vi "Generate Icon.vi"(6 "Access":enum16{"Read", "Write", "R/W"}(ring)=enum."Write", 8 "error in (no error)":errorcluster, 9 "Body":T1={"Line 1 text"="    ", "Line 2 text"="GEN", "Line 3 text"="ICON", "Body text color"=2171169}, 10 "Header":T3={"Header text"="TEST", "Header colors (black, white)"={"Border"=0, "Background"=16730898}, "Header text color"=16777226}, 11 "VI ref":refnum<vi>) -> (0 "error out":errorcluster, 3 "VI ref out":refnum<vi>)   [LabVIEW 2018]
doc: "Generates icon and text for new VI accessors."
uses:
  <vilib>/LabVIEW Icon API/API_Rectangle Colors.ctl
  <vilib>/LabVIEW Icon API/API_Rectangle Dimension.ctl
  <vilib>/LabVIEW Icon API/API_Test Settings.ctl
  <vilib>/LabVIEW Icon API/lv_icon/Controls/Alignment.ctl
  <vilib>/LabVIEW Icon API/API_Text Colors.ctl
  <vilib>/LabVIEW Icon API/API_Text.ctl
  <vilib>/LabVIEW Icon API/API_User Layer Data.ctl
  <vilib>/Utility/miscctls.llb/LVPoint32TypeDef.ctl
  <vilib>/picture/picture.llb/imagedata.ctl
  <vilib>/Utility/error.llb/Clear Errors.vi
  <userlib>/nLight Error Handling/Log any errors.vi
  <vilib>/LabVIEW Icon API/LabVIEW Icon API.lvlib
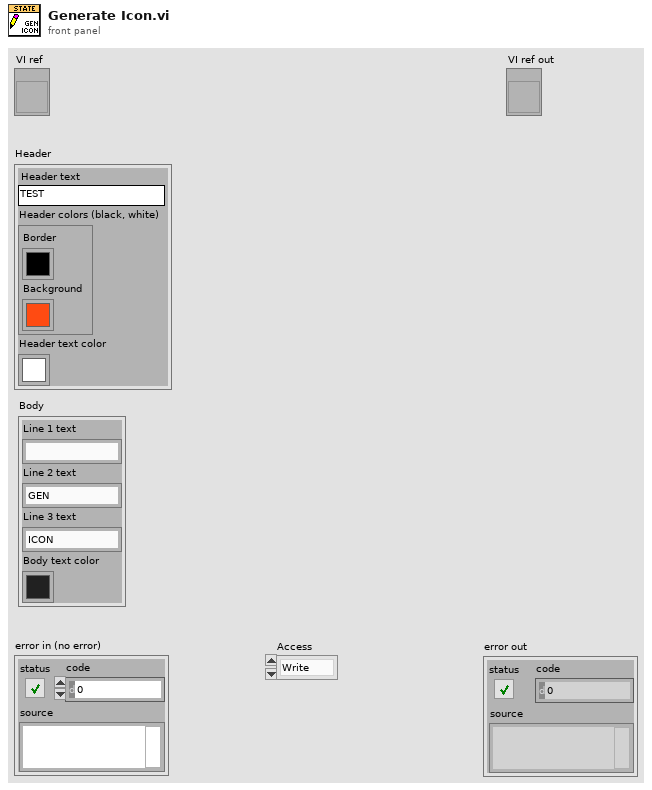
[diagram p1: front panel]
types:
  T1 = cluster{"Line 1 text":string, "Line 2 text":string, "Line 3 text":string, "Body text color":u32}
  T2 = typedef "LabVIEW Icon API.lvlib/API_Rectangle Colors.ctl" = cluster{"Border":u32, "Background":u32}
  T3 = cluster{"Header text":string, "Header colors (black, white)":T2, "Header text color":u32}
  T4 = typedef "Alignment.ctl" = u16
  T5 = typedef "LabVIEW Icon API.lvlib/API_Text.ctl" = cluster{"Line 1 text":string, "Line 2 text":string, "Line 3 text":string, "Line 4 text":string}
  T6 = typedef "LabVIEW Icon API.lvlib/API_Test Settings.ctl" = cluster{"Font":string, "Alignment":T4, "Size":u8, "Center text":bool, "Capitalize text":bool, "Text color":T7}
  T7 = typedef "LabVIEW Icon API.lvlib/API_Text Colors.ctl" = cluster{"Line 1 color":u32, "Line 2 color":u32, "Line 3 color":u32, "Line 4 color":u32}
  T8 = typedef "LabVIEW Icon API.lvlib/API_Rectangle Dimension.ctl" = cluster{"Width":i16, "Height":i16}
  T9 = typedef "imagedata.ctl" = cluster{"image type":i32, "image depth":i32, "image":u8[], "mask":u8[], "colors":u32[], "Rectangle":cluster{"left":i16, "top":i16, "right":i16, "bottom":i16}}
  T10 = typedef "LabVIEW Icon API.lvlib/API_User Layer Data.ctl" = cluster{"Layer name":string, "Origin":T11, "Icon image data":T9}
  T11 = typedef "LVPoint32TypeDef.ctl" = cluster{"Horizontal":i32, "Vertical":i32}
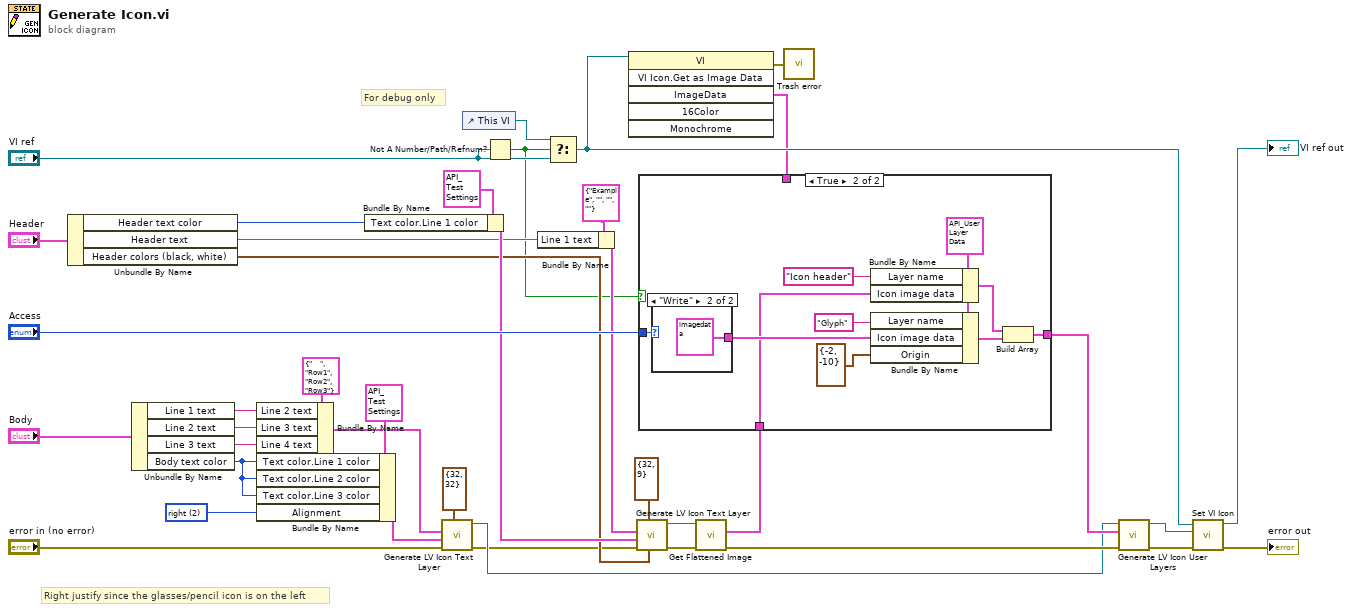
[diagram p0: block diagram]
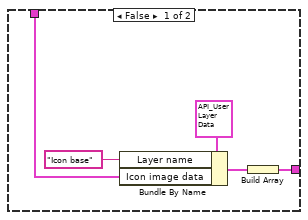
[diagram p2: hidden frame]
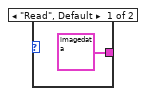
[diagram p3: hidden frame]
diagram:
  w2 = T4 2 items=["left", "center", "right"] ("Alignment")
  # "Right justify since the glasses/pencil icon is on the left"
  # "For debug only"
  n1 = Unbundle By Name("Header") -> ("Header text color"=w20:u32, "Header text"=w19:string, "Header colors (black, white)"=w18:T2)
  n2 = Unbundle By Name("Body") -> ("Line 1 text"=w11:string, "Line 2 text"=w10:string, "Line 3 text"=w9:string, "Body text color"=w16:u32)
  n3 = Bundle By Name(cluster=T5 {"Line 1 text"="    ", "Line 2 text"="Row1", "Line 3 text"="Row2", "Line 4 text"="Row3"} ("Body text"), "Line 2 text"=w11, "Line 3 text"=w10, "Line 4 text"=w9) -> (w12:T5)
  n4 = Bundle By Name(cluster=T6 {"Font"="Small Fonts", "Alignment"=2, "Size"=9, "Center text"=TRUE, "Capitalize text"=TRUE, "Text color"={"Line 1 color"=0, "Line 2 color"=0, "Line 3 color"=0, "Line 4 color"=0}} ("Text settings"), "Text color.Line 1 color"=w16, "Text color.Line 2 color"=w16, "Text color.Line 3 color"=w16, "Alignment"=w2) -> (w24:T6)
  n5 = Bundle By Name(cluster=T6 {"Font"="Small Fonts", "Alignment"=1, "Size"=8, "Center text"=TRUE, "Capitalize text"=TRUE, "Text color"={"Line 1 color"=0, "Line 2 color"=0, "Line 3 color"=0, "Line 4 color"=0}} ("Text settings"), "Text color.Line 1 color"=w20) -> (w26:T6)
  n6 = call <vilib>:"Generate LV Icon Text Layer.vi"("Rectangle dimension (32,32)"=T8 {"Width"=32, "Height"=32}, "error in (no error)"="error in (no error)", "Text settings"=w24, "Text"=w12) -> ("error out"=w14:errorcluster, "Icon out"=w15:refnum<class "Icon.lvclass">)  [unwired: 6 in]
  n7 = control-ref of="This VI"() -> (w7:refnum<vi>)
  n8 = Not A Number/Path/Refnum?(number/path/refnum="VI ref") -> (NaN/Path/Refnum?=w3:bool)
  n9 = Bundle By Name(cluster=T5 {"Line 1 text"="Example", "Line 2 text"="", "Line 3 text"="", "Line 4 text"=""} ("Text"), "Line 1 text"=w19) -> (w28:T5)
  n10 = Select(t=w7, s=w3, f="VI ref") -> (s? t:f=w5:refnum<vi>)
  n11 = invoke class="VI" method="VI Icon.Get as Image Data"(reference=w5) -> (error out=w1:errorcluster, "ImageData"=w4:T9)  [unwired: 5 in, 4 out]
  n12 = call <vilib>:"Generate LV Icon Text Layer.vi"("Rectangle colors (black, white)"=w18, "Rectangle dimension (32,32)"=T8 {"Width"=32, "Height"=9}, "error in (no error)"=w14, "Text settings"=w26, "Text"=w28) -> ("error out"=w30:errorcluster, "Icon out"=w32:refnum<class "Icon.lvclass">)  [unwired: 5 in]
  n13 = call <vilib>:"Get Flattened Image.vi"("error in (no error)"=w30, "lv_icon.lvlib:Icon.lvclass in"=w32) -> ("error out"=w29:errorcluster, "Color Image"=w33:T9)  [unwired: 6 in, 2 out]
  n14 = case shown="True" w3 {
    tunnel: [w41 w53] -> w38
    tunnel: "Access" -> [_ w52]
    tunnel: w33 -> [_ w50]
    tunnel: w4 -> [w40 _]
    frame False {
      n15 = Bundle By Name(cluster=T10 {"Layer name"="", "Origin"={"Horizontal"=0, "Vertical"=0}, "Icon image data"={"image type"=0, "image depth"=0, "image"=[], "mask"=[], "colors"=[], "Rectangle"={"left"=0, "top"=0, "right"=0, "bottom"=0}}} ("User layer"), "Layer name"="Icon base", "Icon image data"=w40) -> (w42:T10)
      n16 = Build Array(w42) -> (w41:T10[])
    }
    frame True {
      w46 = T10 {"Layer name"="", "Origin"={"Horizontal"=0, "Vertical"=0}, "Icon image data"={"image type"=0, "image depth"=0, "image"=[], "mask"=[], "colors"=[], "Rectangle"={"left"=0, "top"=0, "right"=0, "bottom"=0}}} ("User layer")
      n17 = case shown="\"Write\"" w52 {
        tunnel: [T9 {"image type"=0, "image depth"=24, "image"=[255, 255, 255, 255, 255, 255, 255, 255, 255, 255, 255, 255, 255, 255, 255, 0, 0, 0, 0, 0, 0, 255, 255, 255, 255, 255, 255, 255, 255, 255, 255, 255, 255, 255, 255, 255, 255, 255, 255, 0, 0, 0, 0, 0, 0, 255, 255, 255, 255, 255, 255, 255, 255, 255, 255, 255, 255, 255, 255, 255, 0, 0, 0, 255, 255, 255, 255, 255, 255, 0, 0, 0, 255, 255, 255, 255, 255, 255, 255, 255, 255, 255, 255, 255, 0, 0, 0, 255, 255, 255, 255, 255, 255, 0, 0, 0, 255, 255, 255, 255, 255, 255, 255, 255, 255, 0, 0, 0, 255, 255, 255, 255, 255, 255, 255, 255, 255, 0, 0, 0, 255, 255, 255, 255, 255, 255, 255, 255, 255, 0, 0, 0, 255, 255, 255, 255, 255, 255, 255, 255, 255, 0, 0, 0, 255, 255, 255, 255, 255, 255, 0, 0, 0, 0, 0, 0, 255, 255, 255, 255, 255, 255, 255, 255, 255, 255, 255, 255, 255, 255, 255, 255, 255, 255, 0, 0, 0, 0, 0, 0, 255, 255, 255, 255, 255, 255, 255, 255, 255, 255, 255, 255, 255, 255, 255, 0, 0, 0, 255, 255, 255, 255, 255, 255, 0, 0, 0, 255, 255, 255, 0, 0, 0, 0, 0, 0, 255, 255, 255, 0, 0, 0, 255, 255, 255, 0, 255, 255, 0, 0, 0, 255, 255, 255, 255, 255, 255, 255, 255, 255, 0, 0, 0, 255, 255, 255, 255, 255, 255, 0, 255, 255, 0, 255, 255, 0, 0, 0, 255, 255, 255, 255, 255, 255, 0, 0, 0, 255, 255, 255, 255, 255, 255, 255, 255, 255, 0, 255, 255, 0, 0, 0, 255, 255, 255, 255, 255, 255, 0, 0, 0, 0, 255, 255, 255, 255, 255, 0, 255, 255, 0, 214, 214, 0, 0, 0, 255, 255, 255, 255, 255, 255, 0, 0, 0, 0, 255, 255, 255, 255, 255, 0, 255, 255, 0, 214, 214, 0, 0, 0, 255, 255, 255, 255, 255, 255, 255, 255, 255, 0, 0, 0, 0, 255, 255, 0, 255, 255, 0, 0, 0, 255, 255, 255, 255, 255, 255, 255, 255, 255, 255, 255, 255, 0, 0, 0, 0, 255, 255, 0, 214, 214, 0, 0, 0, 255, 255, 255, 255, 255, 255, 255, 255, 255, 255, 255, 255, 255, 255, 255, 0, 0, 0, 0, 0, 0, 255, 255, 255, 255, 255, 255, 255, 255, 255, 255, 255, 255, 255, 255, 255, 255, 255, 255, 0, 0, 0, 0, 0, 0, 255, 255, 255, 255, 255, 255, 255, 255, 255, 255, 255, 255, 255, 255, 255, 255, 255, 255, 255, 255, 255, 255, 255, 255, 255, 255, 255, 255, 255, 255, 255, 255, 255, 255, 255, 255, 255, 255, 255, 255, 255, 255, 255, 255, 255, 255, 255, 255, 255, 255, 255, 255, 255, 255, 255, 255, 255, 255, 255, 255, 255, 255, 255, 255, 255, 255, 255, 255, 255, 255, 255, 255, 255, 255, 255, 255, 255, 255, 255, 255, 255, 255, 255, 255, 255, 255, 255, 255, 255, 255, 255, 255, 255, 255, 255, 255, 255, 255, 255, 255, 255, 255, 255, 255, 255, 255, 255, 255, 255, 255, 255, 255, 255, 255, 255, 255, 255, 255, 255, 255, 255, 255, 255, 255, 255, 255, 255, 255, 255, 255, 255, 255, 255, 255, 255, 255, 255, 255, 255, 255, 255, 255, 255, 255, 255, 255, 255, 255, 255, 255, 255, 255, 255, 255, 255, 255, 255, 255, 255, 255, 255, 255, 255, 255, 255, 255, 255, 255, 255, 255, 255, 255, 255, 255, 255, 255, 255, 255, 255, 255, 255, 255, 255, 255, 255, 255, 255, 255, 255, 255, 255, 255, 255, 255, 255, 255, 255, 255, 255, 255, 255, 255, 255, 255], "mask"=[], "colors"=[], "Rectangle"={"left"=0, "top"=0, "right"=16, "bottom"=13}} ("image subset") T9 {"image type"=0, "image depth"=8, "image"=[0, 0, 0, 0, 1, 1, 1, 1, 0, 0, 0, 0, 0, 0, 1, 3, 3, 3, 1, 0, 0, 0, 0, 1, 3, 3, 3, 3, 1, 0, 0, 0, 0, 1, 1, 3, 3, 1, 0, 0, 0, 0, 1, 2, 2, 1, 1, 1, 0, 0, 0, 0, 1, 2, 2, 2, 1, 0, 0, 0, 0, 1, 2, 2, 2, 2, 1, 0, 0, 0, 0, 1, 2, 2, 2, 1, 0, 0, 0, 0, 1, 2, 2, 2, 2, 1, 0, 0, 0, 0, 1, 2, 2, 2, 1, 0, 0, 0, 0, 0, 1, 1, 2, 2, 1, 0, 0, 0, 0, 0, 1, 1, 1, 1, 0, 0, 0, 0, 0, 0, 1, 1, 1, 0, 0, 0, 0, 0, 0, 0, 1, 1, 0, 0, 0, 0, 0, 0, 0, 0, 1, 0, 0, 0, 0, 0, 0, 0, 0, 0], "mask"=[], "colors"=[16777215, 0, 16776960, 16711935, 0, 0, 0, 0, 0, 0, 0, 0, 0, 0, 0, 0, 0, 0, 0, 0, 0, 0, 0, 0, 0, 0, 0, 0, 0, 0, 0, 0, 0, 0, 0, 0, 0, 0, 0, 0, 0, 0, 0, 0, 0, 0, 0, 0, 0, 0, 0, 0, 0, 0, 0, 0, 0, 0, 0, 0, 0, 0, 0, 0, 0, 0, 0, 0, 0, 0, 0, 0, 0, 0, 0, 0, 0, 0, 0, 0, 0, 0, 0, 0, 0, 0, 0, 0, 0, 0, 0, 0, 0, 0, 0, 0, 0, 0, 0, 0, 0, 0, 0, 0, 0, 0, 0, 0, 0, 0, 0, 0, 0, 0, 0, 0, 0, 0, 0, 0, 0, 0, 0, 0, 0, 0, 0, 0, 0, 0, 0, 0, 0, 0, 0, 0, 0, 0, 0, 0, 0, 0, 0, 0, 0, 0, 0, 0, 0, 0, 0, 0, 0, 0, 0, 0, 0, 0, 0, 0, 0, 0, 0, 0, 0, 0, 0, 0, 0, 0, 0, 0, 0, 0, 0, 0, 0, 0, 0, 0, 0, 0, 0, 0, 0, 0, 0, 0, 0, 0, 0, 0, 0, 0, 0, 0, 0, 0, 0, 0, 0, 0, 0, 0, 0, 0, 0, 0, 0, 0, 0, 0, 0, 0, 0, 0, 0, 0, 0, 0, 0, 0, 0, 0, 0, 0, 0, 0, 0, 0, 0, 0, 0, 0, 0, 0, 0, 0, 0, 0, 0, 0, 0, 0, 0, 0, 0, 0, 0, 0, 0, 0, 0, 0, 0, 0], "Rectangle"={"left"=0, "top"=0, "right"=9, "bottom"=15}} ("image data")] -> w51
        frame "Read", Default {
        }
        frame "Write" {
        }
      }
      n18 = Bundle By Name(cluster=w46, "Layer name"="Icon header", "Icon image data"=w50) -> (w48:T10)
      n19 = Bundle By Name(cluster=w46, "Layer name"="Glyph", "Icon image data"=w51, "Origin"=T11 {"Horizontal"=-2, "Vertical"=-10}) -> (w45:T10)
      n20 = Build Array(w48, w45) -> (w53:T10[])
    }
  }
  n21 = call <userlib>:"Trash error.vi"("error in"=w1) -> ()  [unwired: 15 in]
  n22 = call <vilib>:"Generate LV Icon User Layers.vi"("error in (no error)"=w29, "User layers"=w38, "Icon in"=w15) -> ("error out"=w31:errorcluster, "Icon out"=w37:refnum<class "Icon.lvclass">)  [unwired: 7 in]
  n23 = call <vilib>:"Set VI Icon.vi"("error in (no error)"=w31, "Icon"=w37, "VI Refnum in"=w5) -> ("error out"=→"error out":errorcluster, "VI Refnum out"=→"VI ref out":refnum<vi>)  [unwired: 7 in]
